vi "AKM43L_InitParam8.vi"(0 "PID Loop Period":dbl=0.001 format="%#_13g", 1 "Motor Quantity":i32=8, 3 "error in (no error)":errorcluster) -> (7 "MotorCtrl":refnum<class "MotorControl.lvclass">, 10 "error out":errorcluster)   [LabVIEW 2015, in "AKM43L.lvclass"]
uses:
  AKM43L.lvclass
  MotorControl/MotorControl.lvclass
panel:
  in  "ShaftEncCPR":dbl=2048.0 format="%#_13g"
  in  "Linearity":dbl=1.0 format="%#_13g"
  in  "Beta":dbl=0.8 format="%#_13g"
  in  "PID gain schedule":T1(array[cluster])=[[{"PID gains"={"proportional gain (Kc)"=0.096, "integral time (Ti, min)"=0.00037292, "derivative time (Td, min)"=9.3229e-05}, "max value"=500.0}], [{"PID gains"={"proportional gain (Kc)"=0.078, "integral time (Ti, min)"=0.00024527, "derivative time (Td, min)"=6.1318e-05}, "max value"=500.0}], [{"PID gains"={"proportional gain (Kc)"=0.065, "integral time (Ti, min)"=0.00023706, "derivative time (Td, min)"=5.9264e-05}, "max value"=500.0}], [{"PID gains"={"proportional gain (Kc)"=0.138, "integral time (Ti, min)"=0.00029457, "derivative time (Td, min)"=7.3643e-05}, "max value"=500.0}], [{"PID gains"={"proportional gain (Kc)"=0.03, "integral time (Ti, min)"=0.000783, "derivative time (Td, min)"=0.0002}, "max value"=0.0}], [{"PID gains"={"proportional gain (Kc)"=0.03, "integral time (Ti, min)"=0.000783, "derivative time (Td, min)"=0.0002}, "max value"=0.0}], [{"PID gains"={"proportional gain (Kc)"=0.03, "integral time (Ti, min)"=0.000783, "derivative time (Td, min)"=0.0002}, "max value"=0.0}], [{"PID gains"={"proportional gain (Kc)"=0.03, "integral time (Ti, min)"=0.000783, "derivative time (Td, min)"=0.0002}, "max value"=0.0}]]
  in  "FrictionModel":cluster{"Coeff+":dbl[], "Coeff-":dbl[]}[](array[cluster])=[{"Coeff+"=[-0.12, 0.37], "Coeff-"=[-0.12, 0.37]}, {"Coeff+"=[-0.12, 0.37], "Coeff-"=[-0.12, 0.37]}, {"Coeff+"=[-0.05, 0.37], "Coeff-"=[-0.05, 0.37]}, {"Coeff+"=[-0.05, 0.37], "Coeff-"=[-0.05, 0.37]}, {"Coeff+"=[0.0, 0.37], "Coeff-"=[0.0, 0.37]}, {"Coeff+"=[0.0, 0.37], "Coeff-"=[0.0, 0.37]}, {"Coeff+"=[0.0, 0.37], "Coeff-"=[0.0, 0.37]}, {"Coeff+"=[0.0, 0.37], "Coeff-"=[0.0, 0.37]}]
  in  "MotorConstant(F/V)":dbl=43.0
  in  "Force Rate (N/min)":cluster{"ForceRateLow":dbl, "ForceRateHigh":dbl}={"ForceRateLow"=600.0, "ForceRateHigh"=600000.0} {"ForceRateHigh" format="%#_13g"; "ForceRateLow" format="%#_13g"}
  in  "TransferRatio":dbl=1.0 format="%#_13g"
  in  "output range":cluster{"output high":dbl, "output low":dbl}={"output high"=5.0, "output low"=-0.5}
  in  "setpoint range":cluster{"setpoint high":dbl, "setpoint low":dbl}={"setpoint high"=150.0, "setpoint low"=5.0}
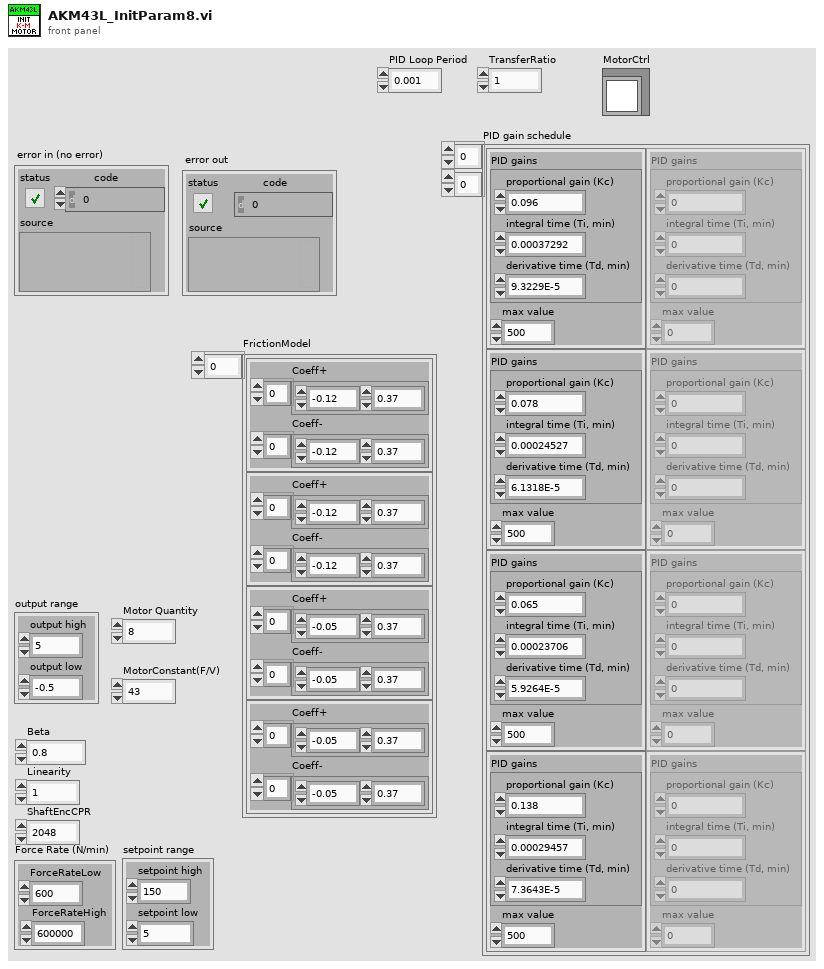
[diagram p1: front panel]
types:
  T1 = cluster{"PID gains":cluster{"proportional gain (Kc)":dbl, "integral time (Ti, min)":dbl, "derivative time (Td, min)":dbl}, "max value":dbl}[][]
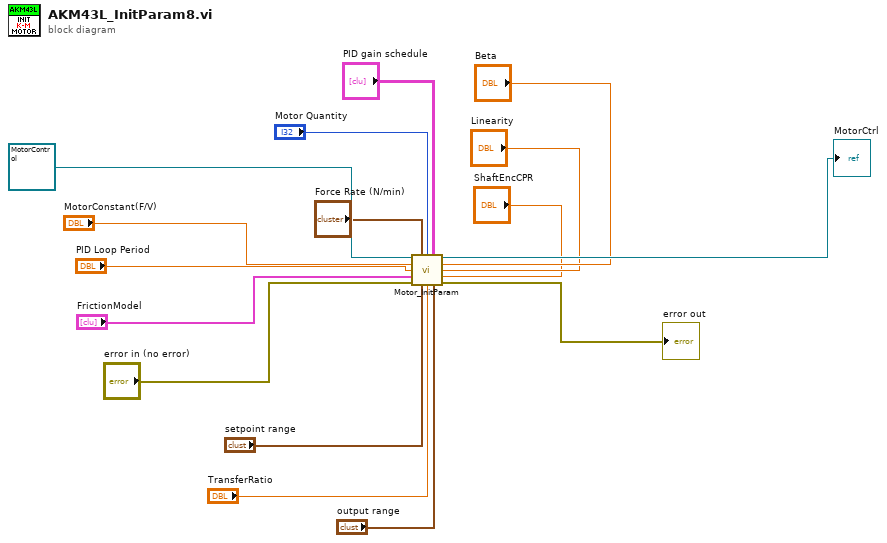
[diagram p0: block diagram]
diagram:
  n1 = call "Motor_InitParam.vi"("Motor Control In"=refnum<class "MotorControl.lvclass"> refnum ("MotorCtrl_In"), "Force Rate Limit (600-10000 N/min)"="Force Rate (N/min)", "Motor Quantity(1)"="Motor Quantity", "PID gain schedule"="PID gain schedule", "MotorConstant(0 F/V)"="MotorConstant(F/V)", "Beta(1)"="Beta", "PID Loop Period(0.001)"="PID Loop Period", "Linearity(1)"="Linearity", "FrictionModel"="FrictionModel", "ShaftEncCPR(1000)"="ShaftEncCPR", "error in (no error)"="error in (no error)", "output range (0 - 100 N)"="setpoint range", "TransferRatio(1)"="TransferRatio", "setpoint range (0 - 1A)"="output range") -> ("Motor Control Out"=→"MotorCtrl":refnum<class "MotorControl.lvclass">, "error out"=→"error out":errorcluster)
